vi "mux_to_alu.vi"(1 "CONTROL":cluster{"c2":bool, "c1":bool, "c0":bool}, 2 "INPUT":T2) -> (0 "OUTPUT":T1)   [LabVIEW 2013]
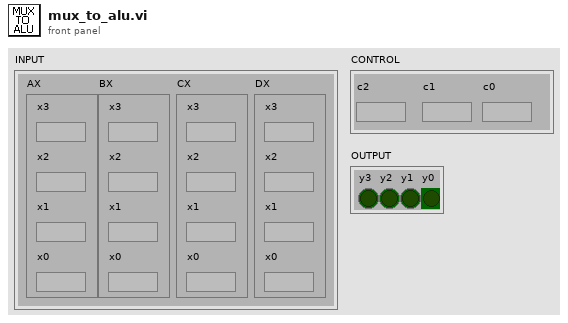
[diagram p1: front panel]
types:
  T1 = cluster{"y3":bool, "y2":bool, "y1":bool, "y0":bool}
  T2 = cluster{"AX":cluster{"x3":bool, "x2":bool, "x1":bool, "x0":bool}, "BX":cluster{"x3":bool, "x2":bool, "x1":bool, "x0":bool}, "CX":cluster{"x3":bool, "x2":bool, "x1":bool, "x0":bool}, "DX":cluster{"x3":bool, "x2":bool, "x1":bool, "x0":bool}}
  T3 = cluster{"x3":bool, "x2":bool, "x1":bool, "x0":bool}
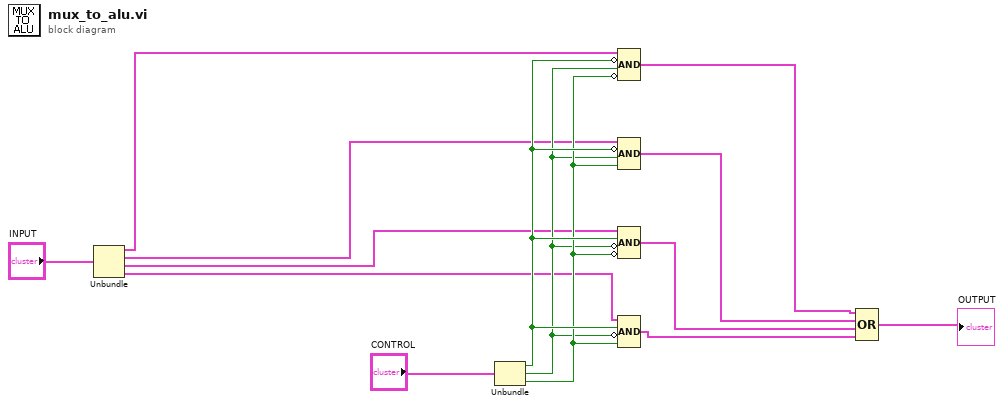
[diagram p0: block diagram]
diagram:
  n1 = Unbundle("INPUT") -> ("AX"=w8:T3, "BX"=w6:T3, "CX"=w5:T3, "DX"=w4:T3)
  n2 = Unbundle("CONTROL") -> ("c2"=w10:bool, "c1"=w7:bool, "c0"=w9:bool)
  n3 = Compound Arithmetic op=AND(w8, invert w10, w7, invert w9) -> (w14:T3)
  n4 = Compound Arithmetic op=AND(w6, invert w10, w7, w9) -> (w13:T3)
  n5 = Compound Arithmetic op=AND(w5, w10, invert w7, invert w9) -> (w12:T3)
  n6 = Compound Arithmetic op=AND(w4, w10, invert w7, w9) -> (w11:T3)
  n7 = Compound Arithmetic op=OR(w14, w13, w12, w11) -> (→"OUTPUT":T3)
